vi "Handle.vi"(8 "error in (no error)":errorcluster, 10 "Zero Timeout Message Handler in":refnum<class "Zero Timeout Message Handler.lvclass">, 11 "Message in":refnum<class "Set Loop Period Msg.lvclass">) -> (0 "error out":errorcluster, 2 "Zero Timeout Message Handler out":refnum<class "Zero Timeout Message Handler.lvclass">)   [LabVIEW 2024, in "PID Loop.lvlib" / "Set Loop Period Msg.lvclass"]
uses:
  src/Zero Timeout Message Handler/Zero Timeout Message Handler/Zero Timeout Message Handler.lvclass
  Set Loop Period Msg.lvclass
  Set Loop Period Msg.lvclass/Set Loop Period Msg.ctl
  PID Loop.lvclass
  C:/Users/uspoaotto/OneDrive - Oregon Tool/Desktop/working copies/zeroTimeoutMessageHandler/src/Zero Timeout Message Handler/Zero Timeout Message Handler/Zero Timeout Message Handler.lvclass
  C:/Users/uspoaotto/OneDrive - Oregon Tool/Desktop/working copies/zeroTimeoutMessageHandler/samples/PID Controller/PID Loop/PID Loop/PID Loop.lvclass
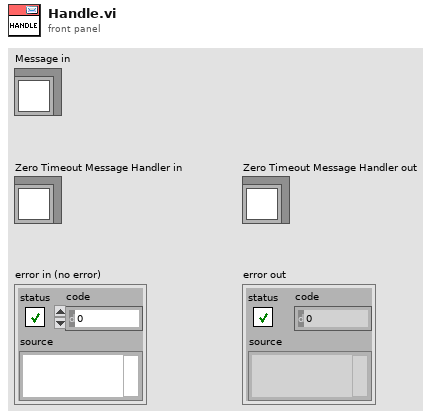
[diagram p1: front panel]
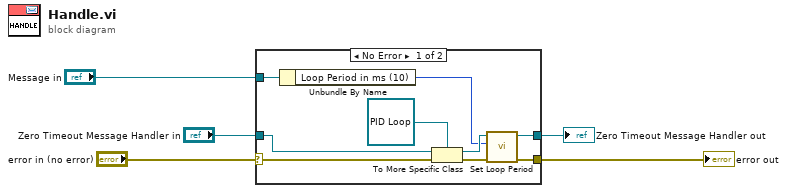
[diagram p0: block diagram]
diagram:
  n1 = case shown="No Error" "error in (no error)" {
    selector: "error in (no error)" -> [w7 w15]
    tunnel: "Zero Timeout Message Handler in" -> [w13 w16]
    tunnel: "Message in" -> [w11 _]
    tunnel: [w9 w15] -> w2
    tunnel: [w6 w16] -> w1
    frame No Error {
      n2 = Unbundle By Name(w11) -> ("Loop Period in ms (10)"=w10:u32)
      n3 = To More Specific Class(target class=refnum<class "PID Loop.lvclass"> refnum ("PID Loop.lvlib:PID Loop.lvclass"), reference=w13, error in=w7) -> (specific class reference=w12:refnum<class "PID Loop.lvclass">, error out=w8:errorcluster)
      n4 = call-dynamic "Set Loop Period.vi"("error in (no error)"=w8, "Loop Period in ms (10)"=w10, "PID Loop in"=w12) -> ("error out"=w9:errorcluster, "PID Loop out"=w6:refnum<class "PID Loop.lvclass">)  [unwired: 7 in]
    }
    frame Error {
    }
  }
  "error out" <- w2
  "Zero Timeout Message Handler out" <- w1
